vi "DialogRenameClass.vi"(0 "ClassWriter.lvclass":refnum<class "ClassWriter.lvclass">, 1 "ClassItemRefIn":refnum<vi>, 5 "error in (no error)":errorcluster) -> (14 "ClassWriter.lvclassOut":refnum<class "ClassWriter.lvclass">, 15 "ClassItemRefOut":refnum<vi>, 16 "NewClassPath":path, 17 "Cancelled":bool, 18 "RelinkWholeProject":bool, 19 "error out":errorcluster)   [LabVIEW 2020, in "ClassWriter.lvclass"]
uses:
  <resource>/Framework/Providers/Open_GDS/ClassProviders/Provider_BaseClassInterface/ClassWriter_class/ClassWriter.lvclass
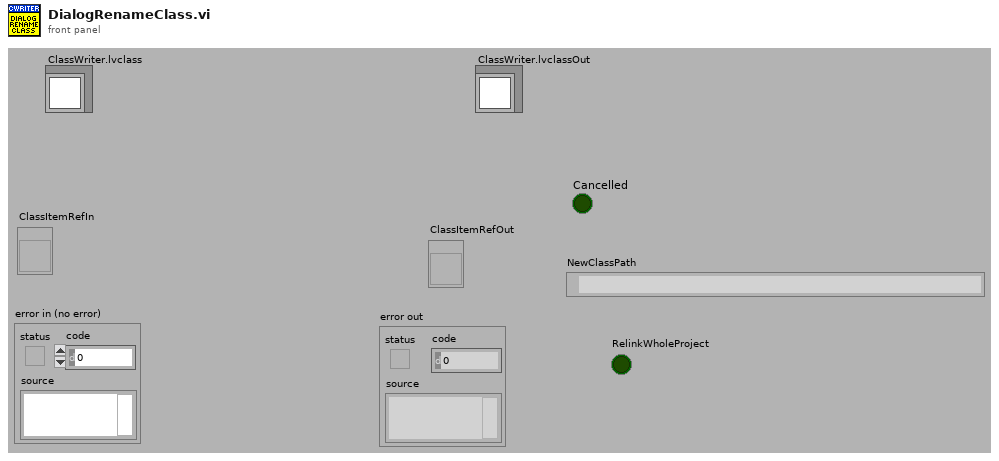
[diagram p1: front panel]
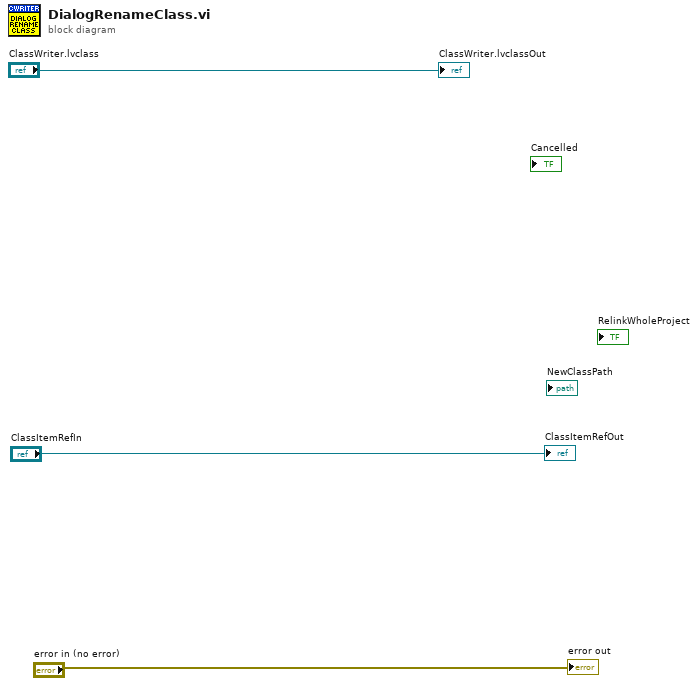
[diagram p0: block diagram]
diagram:
  "ClassItemRefOut" <- "ClassItemRefIn"
  "error out" <- "error in (no error)"
  "ClassWriter.lvclassOut" <- "ClassWriter.lvclass"
